vi "GenerateSquarewaveOutput.vi"(8 "Init":bool, 9 "Duty Cycle (%)":dbl=100.0, 10 "Amplitude":dbl=1.0, 11 "Period (s)":dbl=10.0) -> (3 "Square Wave Ouput":dbl)   [LabVIEW 2020]
doc: "Generates a square wave output with amplitude and period as a function of time"
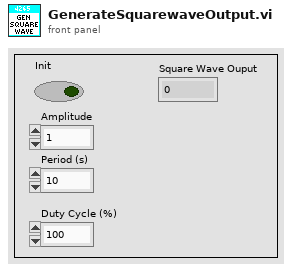
[diagram p1: front panel]
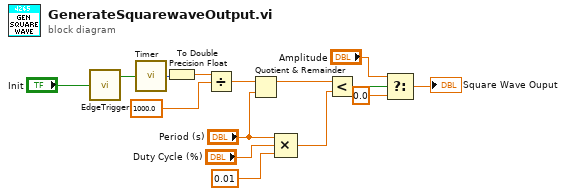
[diagram p0: block diagram]
diagram:
  n1 = call "EdgeTrigger.vi"("Input Signal"="Init") -> ("Rising Edge Trigger"=w15:bool)  [unwired: 2 out]
  n2 = call "Timer.vi"("Reset Timer"=w15) -> ("Time (ms)"=w12:u32)
  n3 = To Double Precision Float(number=w12) -> (double precision float=w13:dbl)
  n4 = Divide(x=w13, y=1000.0) -> (x/y=w10:dbl)
  n5 = Quotient & Remainder(x=w10, y="Period (s)") -> (x-y*floor(x/y)=w9:dbl)  [unwired: 1 out]
  n6 = Compound Arithmetic op=MULTIPLY("Period (s)", "Duty Cycle (%)", 0.01 ("value")) -> (w5:dbl)
  n7 = Less?(x=w9, y=w5) -> (x < y?=w4:bool)
  n8 = Select(t="Amplitude", s=w4, f=0.0) -> (s? t:f=→"Square Wave Ouput":dbl)
